vi "Load Standard.vi"(6 "기준기정렬":u16(ring) items=["등록번호"=0, "기준기명"=1, "형식"=3], 8 "에러 입력(에러 없음)":errorcluster, 10 "선택된 기준기":refnum<vi>, 11 "기준기 리스트":refnum<vi>) -> (0 "에러 출력":errorcluster, 3 "Data out":string[][](array[string]))   [LabVIEW 2020]
uses:
  Controls/Cmd_Select Setting.ctl
  Controls/Cmd_Read Query.ctl
  Controls/Clst_Query Info.ctl
  Variables/Global_Cal Info.vi
  Public/Polymorph/Array Dedup_2D Str.vi
  Public/Polymorph/Sort_2D Str.vi
  Public/Polymorph/Cell Space_ListBox.vi
  Variables/Global_Cal STD.vi
  <vilib>/addons/database/NI_Database_API.lvlib
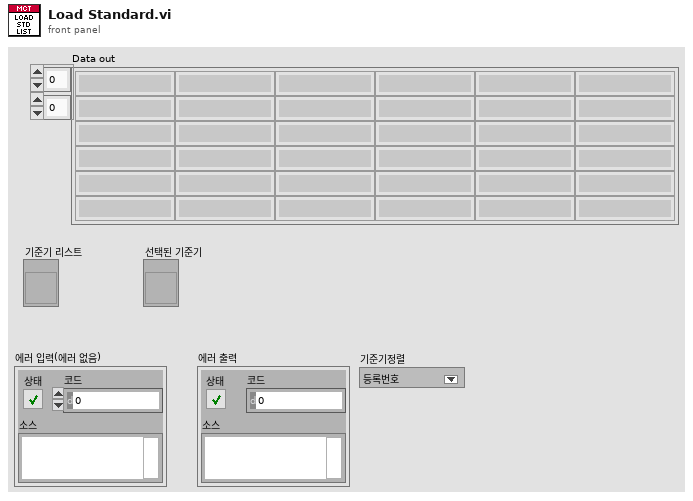
[diagram p1: front panel]
types:
  T1 = typedef "Cmd_Select Setting.ctl" = enum16{"STD Setting"}
  T2 = cluster{"세부분류코드":string, "형식":string, "옵션":string, "측정기명":string, "EXCEL파일명":string, "TEMP":string}
  T3 = typedef "NI_Database_API.lvlib/Conn ObjectReference.ctl" = refnum<k1>
  T4 = typedef "Clst_Query Info.ctl" = cluster{"사번":string, "등록번호":string, "업체명":string, "세부분류코드":string, "형식":string, "기기번호":string, "FUNC":string, "FUNC_EXT":string, "옵션":string, "추가문자열":string, "일자":string, "배열 1":string[], "배열 2":string[], "항목명":string, "문자열":string, "이름":string}
  T5 = typedef "Cmd_Read Query.ctl" = enum16{"교정자 이름 얻기", "인증교정자 얻기", "기술책임자 얻기", "기책부책 얻기", "등록번호 얻기", "등록정보 얻기", "업체정보 얻기", "교정일자(CAMAS) 얻기", "교정일자(CALSTD) 얻기", "교정환경 얻기", "교정절차서 목록 얻기", "교정절차서명 얻기", "교정절차 목록얻기", "교정절차 얻기", "PROC 교정절차 얻기", "PROC SPEC 얻기", "교정절차(Func별) 얻기", "교정절차(Func_ext별) 얻기", "기관코드 얻기", "교정기능(세부분류) 얻기", "교정기능(모델) 얻기", "교정기능 목록 얻기", "교정기능 명칭 얻기", "교정기능 항목명칭 얻기", "DB (사용기준기) 얻기", "DB (기준기이름) 얻기", "DB (기준기이름목록) 얻기", "DB (기준기목록) 얻기", "DB (기준기값) 얻기", "DB (CMC) 얻기", "DB (FUNC) 얻기", "DB (CALNAME) 얻기", "DB (STDNAME) 얻기", "DB (SPEC) 얻기", "모델(항목전체) 얻기", "모델(최대범위) 얻기", "모델(최소범위) 얻기", "모델(최대최소) 얻기", "모델(범위조건) 얻기", "모델(등록요청) 얻기", "모델(형식별) 얻기", "모델(조건별) 얻기", "모델(모델검색) 얻기", "세부분류 목록 얻기", "기준기등록리스트 얻기", "STD Cal Date Check", "DB등록일자 얻기", "적용항목 얻기", "기타정보 얻기", "기준기요청 얻기", "서버버전 얻기"}
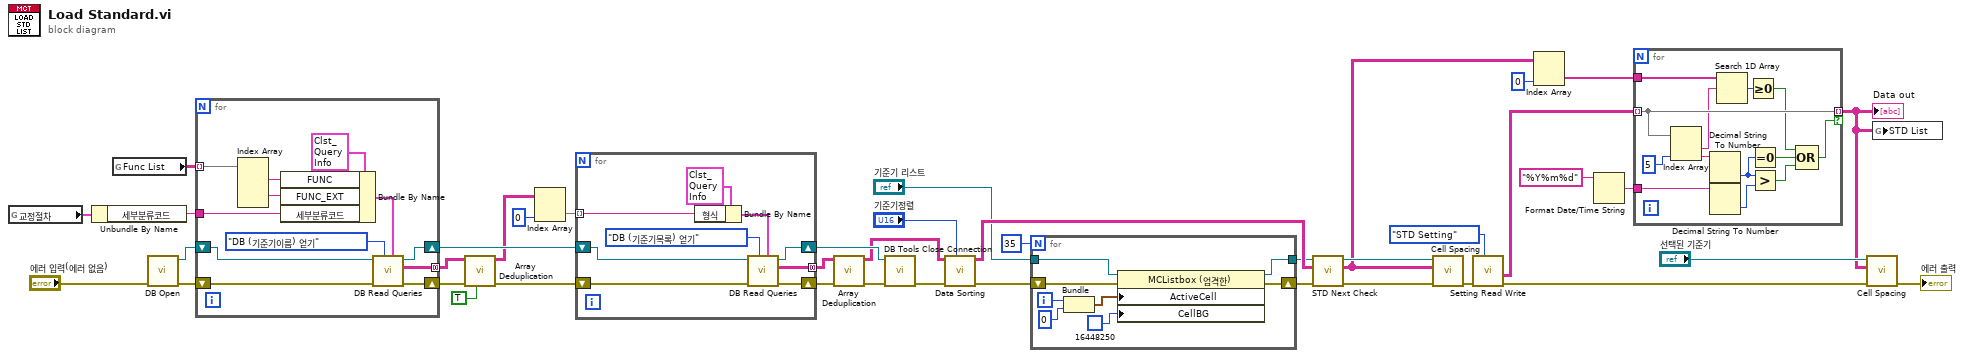
[diagram p0: block diagram]
diagram:
  n1 = global read "Global_Cal Info.vi" "교정절차"() -> (w9:T2)
  n2 = Unbundle By Name(w9) -> ("세부분류코드"=w8:string)
  n3 = global read "Global_Cal Info.vi" "Func List"() -> (w28:string[][])
  n4 = call "DB Open.vi"("에러 입력"="에러 입력(에러 없음)") -> ("에러 출력"=w39:errorcluster, "참조 번호 출력"=w40:T3)  [unwired: 9 in]
  n5 = for {
    shift-right: [w49] -> w37
    shift-left: w39 -> [w52]
    tunnel: w28 -> [w47] mode=indexing
    shift-right: [w50] -> w36
    shift-left: w40 -> [w51]
    tunnel: [w42] -> w33 mode=concatenating
    tunnel: w8 -> [w41]
    n6 = Index Array(array=w47) -> (element #1=w45:string, element #3=w44:string)  [unwired: 4 in, 2 out]
    n7 = Bundle By Name(cluster=T4 {"사번"="", "등록번호"="", "업체명"="", "세부분류코드"="", "형식"="", "기기번호"="", "FUNC"="", "FUNC_EXT"="", "옵션"="", "추가문자열"="", "일자"="", "배열 1"=[], "배열 2"=[], "항목명"="", "문자열"="", "이름"=""} ("Query info"), "FUNC"=w45, "FUNC_EXT"=w44, "세부분류코드"=w41) -> (w43:T4)
    n8 = call "DB Read Queries.vi"("Query info"=w43, "Query Command"=Cmd_Read_Query."DB (기준기이름) 얻기", "에러 입력(에러 없음)"=w52, "참조 번호 입력"=w51) -> ("에러 출력"=w49:errorcluster, "Data"=w42:string[][], "참조 번호 출력"=w50:T3)  [unwired: 3 in, 2 out]
  }
  n9 = call-poly "Array Deduplication.vi"("정렬?"=TRUE, "error in (no error)"=w37, "배열 in"=w33) -> ("error out"=w34:errorcluster, "배열 out"=w31:string[][])  [unwired: 7 in]
  n10 = Index Array(array=w31, index (col)=0 ("비활성화된 인덱스 (열)")) -> (element=w30:string[])  [unwired: 1 in]
  n11 = for {
    shift-right: [w60] -> w27
    shift-left: w34 -> [w61]
    shift-right: [w58] -> w35
    shift-left: w36 -> [w59]
    tunnel: w30 -> [w53] mode=indexing
    tunnel: [w54] -> w25 mode=concatenating
    n12 = Bundle By Name(cluster=T4 {"사번"="", "등록번호"="", "업체명"="", "세부분류코드"="", "형식"="", "기기번호"="", "FUNC"="", "FUNC_EXT"="", "옵션"="", "추가문자열"="", "일자"="", "배열 1"=[], "배열 2"=[], "항목명"="", "문자열"="", "이름"=""} ("Query info"), "형식"=w53) -> (w55:T4)
    n13 = call "DB Read Queries.vi"("Query info"=w55, "Query Command"=Cmd_Read_Query."DB (기준기목록) 얻기", "에러 입력(에러 없음)"=w61, "참조 번호 입력"=w59) -> ("에러 출력"=w60:errorcluster, "Data"=w54:string[][], "참조 번호 출력"=w58:T3)  [unwired: 3 in, 2 out]
  }
  n14 = call-poly "Array Deduplication.vi"("error in (no error)"=w27, "배열 in"=w25) -> ("error out"=w26:errorcluster, "배열 out"=w20:string[][])  [unwired: 8 in]
  n15 = call <vilib>:"DB Tools Close Connection.vi"("error in (no error)"=w26, "connection reference"=w35) -> ("error out"=w21:errorcluster)  [unwired: 5 in]
  n16 = call-poly "Data Sorting.vi"("기준열"="기준기정렬", "error in (no error)"=w21, "Data in"=w20) -> ("error out"=w7:errorcluster, "Data out"=w19:string[][])  [unwired: 7 in]
  n17 = for {
    N: 35 -> [_]
    shift-right: [w68] -> _
    shift-left: w7 -> [w69]
    tunnel: "기준기 리스트" -> [w67]
    tunnel: [w62] -> w4
    i -> [w64]
    n18 = Bundle(w64, 0) -> (w65:cluster{i32, i32})  [unwired: 1 in]
    n19 = property class="MCListbox (엄격한)"(reference=w67, error in=w69, "ActiveCell"=w65, "CellBG"=u32 16448250) -> (reference out=w62:refnum<vi>, error out=w68:errorcluster)
  }
  n20 = call "STD Next Check.vi"("에러 입력"=w7, "Data in"=w19, "기준기리스트 참조 입력"=w4) -> ("에러 출력"=w24:errorcluster, "Data out"=w3:string[][], "기준기리스트 참조 출력"=w23:refnum<vi>)  [unwired: 6 in]
  n21 = call-poly "Cell Spacing.vi"("error in"=w24, "Data in"=w3, "여러열리스트박스 참조 in"=w23) -> ("error out"=w13:errorcluster)  [unwired: 7 in, 1 out]
  n22 = call "Setting Read Write.vi"("Select"=Cmd_Select_Setting."STD Setting", "error in (no error)"=w13) -> ("error out"=w12:errorcluster, "Data out"=w14:string[][])  [unwired: 8 in]
  n23 = Index Array(array=w3, index (col)=0 ("비활성화된 인덱스 (열)")) -> (element=w1:string[])  [unwired: 1 in]
  n24 = Format Date/Time String(time format string (%c)="%Y%m%d" ("시간 포맷 문자열 (%c)")) -> (date/time string=w16:string)  [unwired: 2 in]
  n25 = for {
    tunnel: w14 -> [w78] mode=indexing
    tunnel: w16 -> [w80]
    tunnel: [w78] -> w10 mode=indexing if=w76
    tunnel: w1 -> [w73]
    n26 = Index Array(array=w78, index #2=5 ("인덱스")) -> (element #1=w72:string, element #2=w81:string)  [unwired: 1 in]
    n27 = Decimal String To Number(string=w81) -> (number=w75:i32)  [unwired: 2 in, 1 out]
    n28 = Decimal String To Number(string=w80) -> (number=w79:i32)  [unwired: 2 in, 1 out]
    n29 = Search 1D Array(1D array=w73, element=w72) -> (index of element=w71:i32)  [unwired: 1 in]
    n30 = Greater Or Equal To 0?(x=w71) -> (x >= 0?=w70:bool)
    n31 = Equal To 0?(x=w75) -> (x = 0?=w74:bool)
    n32 = Greater?(x=w75, y=w79) -> (0:w77:bool)
    n33 = Compound Arithmetic op=OR ("복합 연산")(w70, w74, w77) -> (w76:bool)
  }
  "Data out" <- w10
  n34 = call-poly "Cell Spacing.vi"("error in"=w12, "Data in"=w10, "여러열리스트박스 참조 in"="선택된 기준기") -> ("error out"=→"에러 출력":errorcluster)  [unwired: 7 in, 1 out]
  n35 = global write "Global_Cal STD.vi" "STD List"(w10) -> ()
